vi "SharedPowersArray.vi"(1 "Write?":bool, 2 "PowersInput":i16[](array[numeric])) -> (0 "Powers":i16[](array[numeric]))   [LabVIEW 2010, in "Player.lvlib"]
uses:
  Player.lvlib
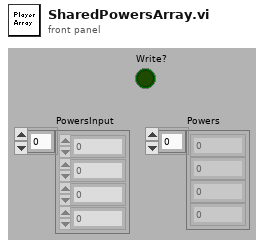
[diagram p1: front panel]
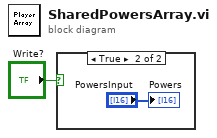
[diagram p0: block diagram]
diagram:
  n1 = case shown="True" "Write?" {
    frame False {
    }
    frame True {
      "Powers" <- "PowersInput"
    }
  }
